vi "Read State.vi"(8 "error in":errorcluster, 11 "Context in":refnum<class "Context.lvclass">) -> (0 "error out":errorcluster, 2 "State":refnum<class "State Pattern.lvclass">, 3 "Context out":refnum<class "Context.lvclass">)   [LabVIEW 2021, in "Context.lvlib" / "Context.lvclass"]
uses:
  Context.lvclass
  State Pattern/State Pattern/State Pattern.lvclass
  Context.lvclass/Context.ctl
  State/State.lvclass
  C:/PPLs/Design-Patterns/State Pattern/State Pattern/State Pattern/State Pattern.lvclass
  C:/PPLs/Design-Patterns/State Pattern/State Pattern/State Change Core/State Change Core/State Change Core.lvclass
  C:/PPLs/Design-Patterns/State Pattern/Example/Context/State/State.lvclass
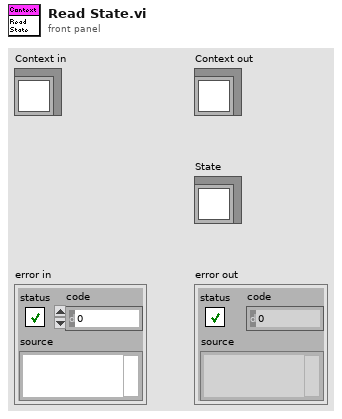
[diagram p1: front panel]
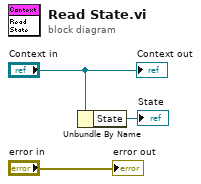
[diagram p0: block diagram]
diagram:
  n1 = Unbundle By Name("Context in") -> ("State"=→"State":refnum<class "State.lvclass">)
  "error out" <- "error in"
  "Context out" <- "Context in"
